vi "getFlags.vi"(11 "UNSUBSCRIBE in":refnum<class "UNSUBSCRIBE.lvclass">) -> (0 "RETAIN":bool, 1 "QoS":T1, 2 "DUP":bool, 3 "UNSUBSCRIBE out":refnum<class "UNSUBSCRIBE.lvclass">)   [LabVIEW 2013, in "MQTT_Control_Packets.lvlib" / "UNSUBSCRIBE.lvclass"]
uses:
  UNSUBSCRIBE.lvclass
  ControlPacket/QualityOfService -- enum.ctl
  ControlPacket/ControlPacket.lvclass
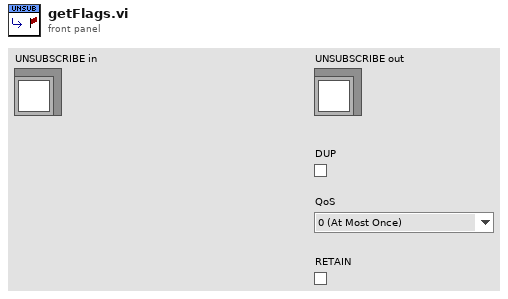
[diagram p1: front panel]
types:
  T1 = typedef "MQTT_Control_Packets.lvlib/ControlPacket.lvclass/QualityOfService -- enum.ctl" = enum16{"0 (At Most Once)", "1 (At Least Once)", "2 (Exactly Once)"}
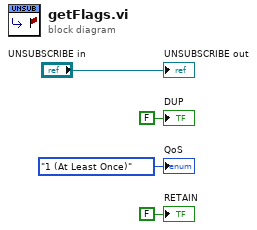
[diagram p0: block diagram]
diagram:
  "UNSUBSCRIBE out" <- "UNSUBSCRIBE in"
  "QoS" <- QualityOfService_--_enum."1 (At Least Once)" ("QoS")
  "DUP" <- FALSE ("DUP")
  "RETAIN" <- FALSE ("RETAIN")
